vi "behavior_only.vi"() -> ()   [LabVIEW 2019]
doc: "The myRIO Project template acquires acceleration data from the onboard accelerometer and displays the changes of acceleration values in a waveform chart."
uses:
  <vilib>/myRIO/Common/Instrument Driver Framework/Utilities/typedefs/Generic FPGA Reference.ctl
  <vilib>/myRIO/Common/Instrument Driver Framework/Utilities/typedefs/myRIO v1.0 Reference.ctl
  <vilib>/myRIO/Common/Instrument Driver Framework/Utilities/typedefs/Hardware Version Enum.ctl
  <vilib>/myRIO/Common/Instrument Driver Framework/Utilities/typedefs/myRIO Generic Hardware Reference.ctl
  <vilib>/userdefined/High Color/nirio_resource_hc.ctl
  <vilib>/myRIO/Common/Instrument Driver Framework/Utilities/vis/Is FPGA Ref Available.vi
  <vilib>/myRIO/Common/Instrument Driver Framework/myRIO v1.0/Encoder/typedefs/Encoder Signal Mode.ctl
  <vilib>/myRIO/Common/Instrument Driver Framework/myRIO v1.0/Encoder/typedefs/Encoder Channels Enum.ctl
  <vilib>/myRIO/Instrument Drivers/Onboard IO/Encoder/typedefs/Encoder Reference.ctl
  <vilib>/myRIO/Instrument Drivers/Onboard IO/Encoder/Encoder.lvlib
  <vilib>/myRIO/Instrument Drivers/Onboard IO/Encoder/vis/Read.vi
  <vilib>/myRIO/Common/Instrument Driver Framework/myRIO v1.0/Encoder/typedefs/Encoder Configuration v1.0.ctl
  <vilib>/myRIO/Common/Instrument Driver Framework/myRIO v1.0/Encoder/vis/myRIO v1.1 Open Encoder.vi
  <vilib>/myRIO/Common/Instrument Driver Framework/myRIO v1.0/Encoder/vis/myRIO v1.0 Configure Encoder.vi
  <vilib>/myRIO/Instrument Drivers/Onboard IO/Encoder/vis/myRIO Encoder Open.xnode
  <vilib>/myRIO/Express VI/Onboard IO/Encoder/Encoder Express VI.xnode
  <vilib>/myRIO/Common/Instrument Driver Framework/myRIO v1.0/Encoder/typedefs/Encoder Count Direction Enum.ctl
panel:
  out "Stop":bool
  in  "Frames to collect":u32
  out "Time":dbl
  out "Frame clock":i32
  out "Overflow?":bool
  out "Counter Value":i32
  out "Velocity":dbl
  out "Velocity Plot":dbl[](graph)
  out "Velocity array":dbl[](array[numeric])
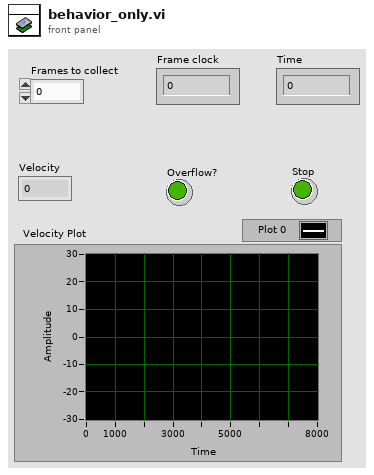
[diagram p1: front panel]
types:
  T1 = typedef "Encoder.lvlib/Encoder Reference.ctl" = cluster{"myRIO Reference":T2, "Encoder Channels Enum":T6}
  T2 = typedef "myRIO Generic Hardware Reference.ctl" = cluster{"myRIO Model":T3, "myRIO Hardware Reference":T4}
  T3 = typedef "Hardware Version Enum.ctl" = enum16{"Unknown", "myRIO-1900", "myRIO-1950", "roboRIO", "NI ELVIS RIO CM", "ELVIS III"}
  T4 = typedef "myRIO v1.0 Reference.ctl" = cluster{"Generic FPGA Reference":T5, "Allow multiple opens":bool}
  T5 = typedef "Generic FPGA Reference.ctl" = refnum<k20>
  T6 = typedef "Encoder Channels Enum.ctl" = enum16{"Not Connected", "C/ENC0", "C/ENC1", "A/ENC", "A/ENC0", "A/ENC1", "A/ENC2", "A/ENC3", "A/ENC4", "A/ENC5", "A/ENC6", "A/ENC7", "A/ENC8", "A/ENC9", "B/ENC", "B/ENC0", "B/ENC1", "B/ENC2", "B/ENC3", "B/ENC4", "B/ENC5", "B/ENC6", "B/ENC7", "B/ENC8", "B/ENC9", "DIO/ENC0", "DIO/ENC1", "DIO/ENC2", "DIO/ENC3", "DIO/ENC4"}
  T7 = typedef "Encoder Signal Mode.ctl" = enum16{"Quadrature phase signal", "Step and direction signal"}
  T8 = typedef "nirio_resource_hc.ctl" = tag
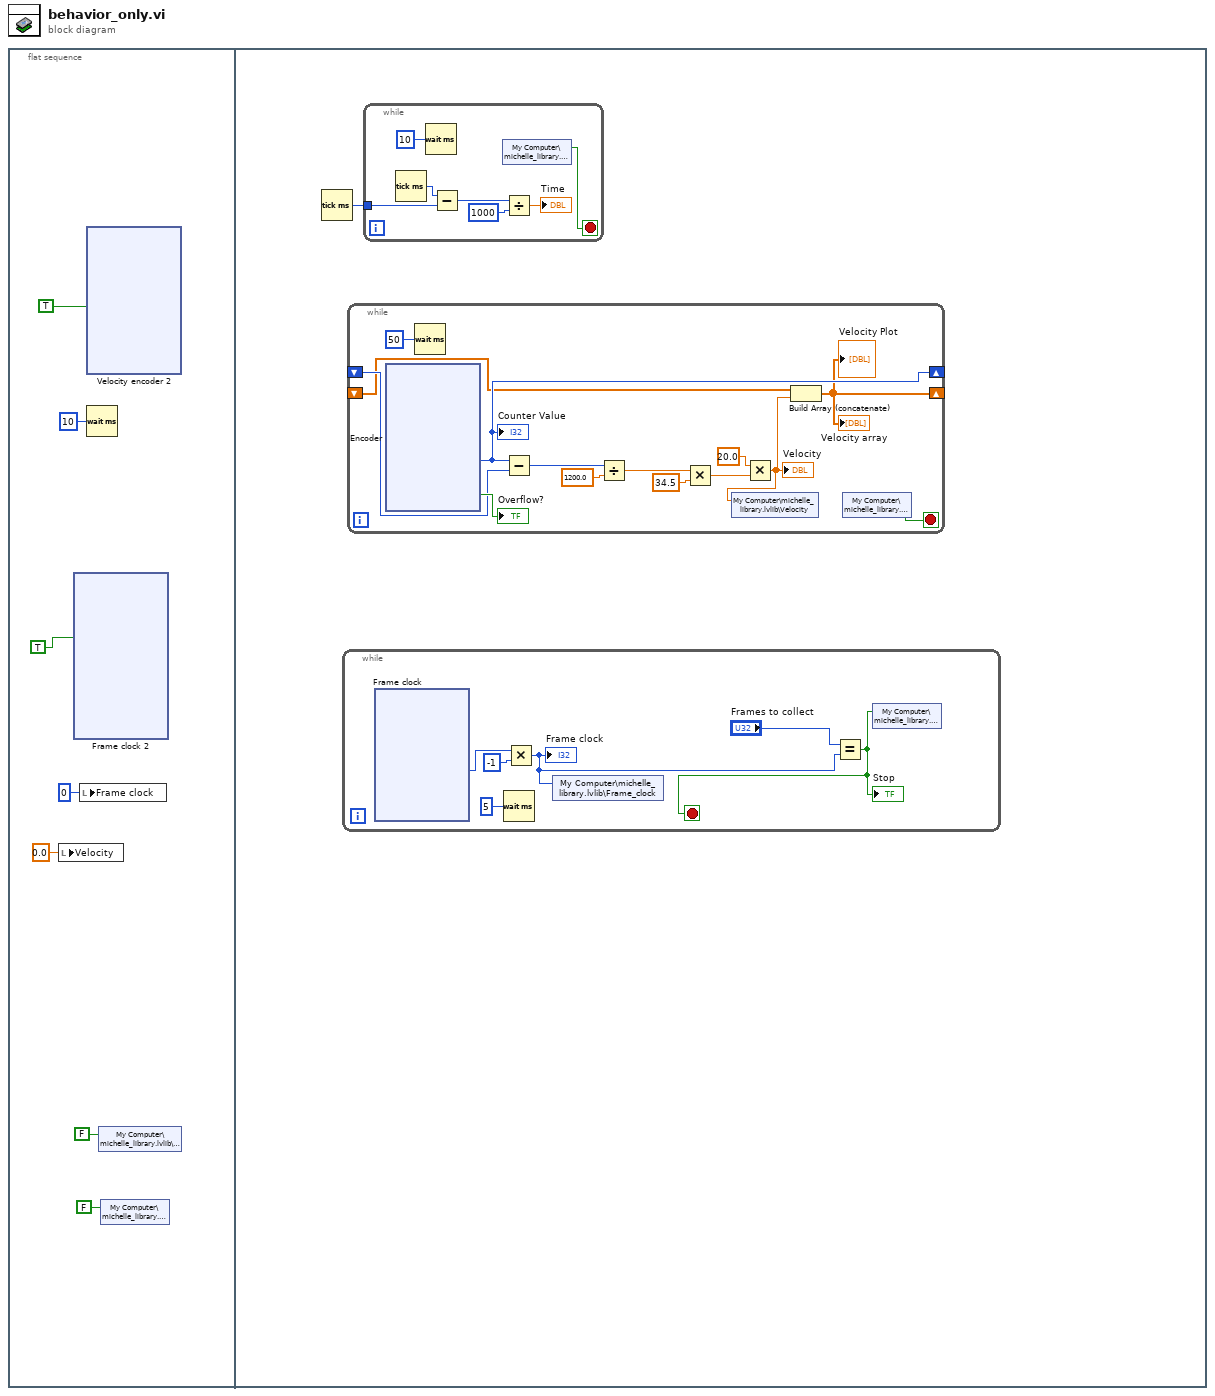
[diagram p0: block diagram]
diagram:
  n1 = flat-sequence {
    frame #0 {
      n2 = local write "Velocity"(0.0 ("Velocity")) -> ()
      n3 = xnode "Frame clock 2"("Reset Counter"=TRUE) -> ()  [unwired: 1 in, 4 out]
      n4 = local write "Frame clock"(0 ("Frame clock")) -> ()
      n5 = xnode "Velocity encoder 2"("Reset Counter"=TRUE) -> ()  [unwired: 1 in, 4 out]
      n6 = Wait (ms)(milliseconds to wait=u32 10) -> ()  [unwired: 1 out]
      n7 = shared-variable "My Computer\\michelle_library.lvlib\\Display"(FALSE ("Display")) -> ()  [unwired: 1 in, 1 out]
      n8 = shared-variable "My Computer\\michelle_library.lvlib\\Stop"(FALSE ("Stop")) -> ()  [unwired: 1 in, 1 out]
    }
    frame #1 {
      n9 = Tick Count (ms)() -> (millisecond timer value=w100:u32)
      n10 = while {
        stop <- w161 stop-if-true
        n11 = xnode "Frame clock"() -> ("Counter Value"=w165:i32)  [unwired: 2 in, 3 out]
        n12 = Wait (ms)(milliseconds to wait=u32 5) -> ()  [unwired: 1 out]
        n13 = Multiply(x=w165, y=-1) -> (x*y=w162:i32)
        "Frame clock" <- w162
        n14 = shared-variable "My Computer\\michelle_library.lvlib\\Frame_clock"(w162) -> ()  [unwired: 1 in, 1 out]
        n15 = Equal?(x="Frames to collect", y=w162) -> (x = y?=w161:bool)
        "Stop" <- w161
        n16 = shared-variable "My Computer\\michelle_library.lvlib\\Stop"(w161) -> ()  [unwired: 1 in, 1 out]
      }
      n17 = while {
        shift-right: [w111] -> _
        shift-left: _ -> [w112]
        shift-right: [w104] -> _
        shift-left: _ -> [w103]
        stop <- w102 stop-if-true
        n18 = xnode "Encoder"() -> ("Counter Value"=w111:i32, "Overflow?"=→"Overflow?":bool)  [unwired: 2 in, 2 out]
        "Counter Value" <- w111
        n19 = Wait (ms)(milliseconds to wait=u32 50) -> ()  [unwired: 1 out]
        n20 = Subtract(x=w111, y=w112) -> (x-y=w105:i32)
        n21 = Divide(x=w105, y=1200.0 ("600")) -> (x/y=w109:dbl)
        n22 = Multiply(x=w109, y=34.5) -> (x*y=w107:dbl)
        n23 = Multiply(x=20.0, y=w107) -> (x*y=w101:dbl)
        "Velocity" <- w101
        n24 = shared-variable "My Computer\\michelle_library.lvlib\\Velocity"(w101) -> ()  [unwired: 1 in, 1 out]
        n25 = Build Array (concatenate)(w103, w101) -> (w104:dbl[])
        "Velocity Plot" <- w104
        "Velocity array" <- w104
        n26 = shared-variable "My Computer\\michelle_library.lvlib\\Stop"() -> (w102:bool)  [unwired: 1 in, 1 out]
      }
      n27 = while {
        tunnel: w100 -> [w218]
        stop <- w213 stop-if-true
        n28 = Tick Count (ms)() -> (millisecond timer value=w219:u32)
        n29 = Wait (ms)(milliseconds to wait=u32 10) -> ()  [unwired: 1 out]
        n30 = Subtract(x=w219, y=w218) -> (x-y=w216:u32)
        n31 = shared-variable "My Computer\\michelle_library.lvlib\\Stop"() -> (w213:bool)  [unwired: 1 in, 1 out]
        n32 = Divide(x=w216, y=u32 1000) -> (x/y=→"Time":dbl)
      }
    }
  }
